vi "fpga.sandbox.test.vi"() -> ()   [LabVIEW 2020]
uses:
  <vilib>/rvi/LocalResourceManager/LocalResourceManager.xnode
  <vilib>/rvi/eio/common/nirviEmuReportErrorAndStop.vi
  <vilib>/rvi/DataTransferAndStorage/Container/Common/niFpgaContainerGetUniqueNameForEmu.vi
  <vilib>/rvi/DataTransferAndStorage/Container/Common/niFpgaContainerSetEmuInfo.vi
  <vilib>/Platform/TimedLoop/XDataNode/wakeup.ctl
  <vilib>/Platform/TimedLoop/XDataNode/XDNodeRunTimeDep.lvlib
  <vilib>/Platform/TimedLoop/XDataNode/nitl_modes.ctl
  <vilib>/Platform/TimedLoop/XDataNode/timing_clust.ctl
  <vilib>/Platform/TimedLoop/XDataNode/XDataNode.xnode
  axi_2_eth_raw.ctl
  <vilib>/rvi/DataTransferAndStorage/Container/XNode/niFpgaContainer.xnode
  <vilib>/rvi/interface/RandomDataEmulation/nirviRandomDataFpgaMultiElementTemplate.vi
  <vilib>/rvi/Memory/Memory_Emulation/niFpgaMemoryEmulationRefIn.vi
  <vilib>/rvi/FIFO/Fifo_Resource/niFpgaFifoEmulationRefIn.vi
  submodules/Market.Data.Bats.Parser/fpga/poc.ip.axi.write.states.ctl
panel:
  in  "ip.Reset":bool
  in  "Reset":bool
  out "Data":T1
  out "i":u16
  out "Numeric":i32
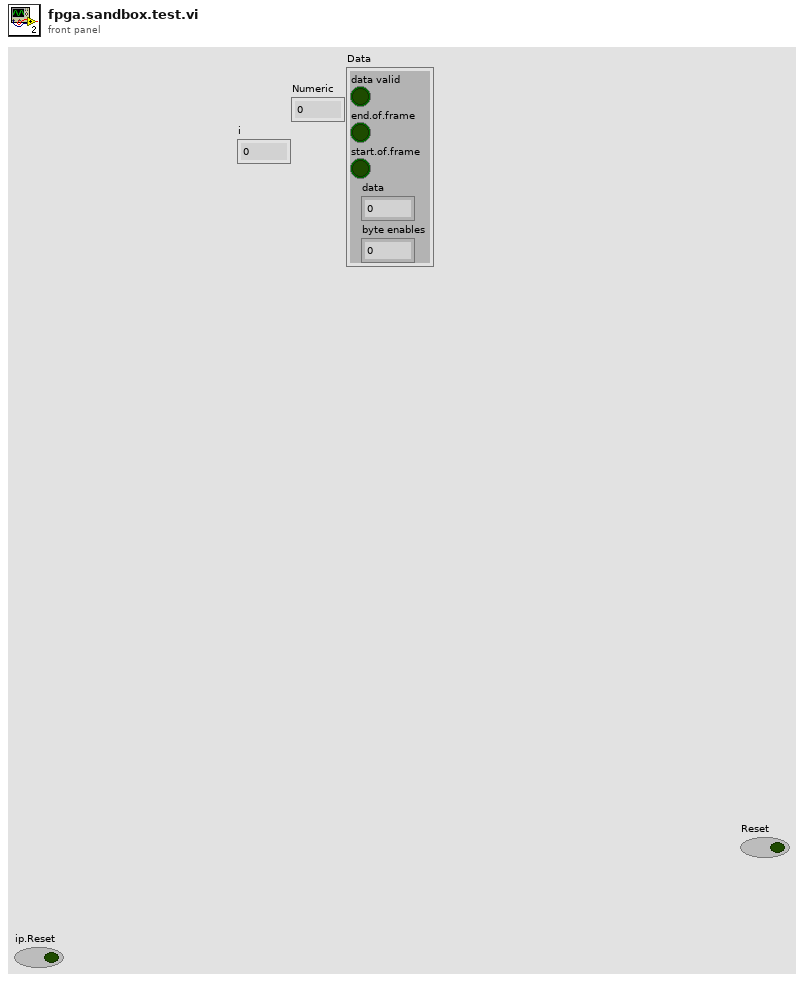
[diagram p1: front panel]
types:
  T1 = cluster{"data valid":bool, "end.of.frame":bool, "start.of.frame":bool, "data":u64, "byte enables":u8}
  T2 = typedef "XDNodeRunTimeDep.lvlib/timing_clust.ctl" = cluster{"Expected End [f-1]":u64, "Actual End [f-1]":u64, "Finished Late? [f-1]":bool, "Expected End [i-1]":u64, "Actual End [i-1]":u64, "Finished Late? [i-1]":bool, "Expected Start [i]":u64, "Actual Start [i]":u64, "Expected Start [f]":u64, "Actual Start [f]":u64, "Source Name":string, "Structure Name":string, "Period":i64, "Deadline":i64, "Offset":i64, "Start":i64, "Priority":i32, "Timeout":i32, "Mode":T3, "Wakeup Reason":T4, "Error":errorcluster, "Source Type":string, "Secondary Source Type":string, "Global End Time":u64, "Global Start Time":u64, "Frame Duration":u64, "Iteration Duration":u64, "Assigned CPU":i32, "I/O Scan Engine Mode":u32}
  T3 = typedef "XDNodeRunTimeDep.lvlib/nitl_modes.ctl" = enum32{"No Change", "Process missed periods, maintain original phase", "Discard missed periods, maintain original phase", "Process missed periods, ignore original phase", "Discard missed periods, ignore original phase"}
  T4 = typedef "XDNodeRunTimeDep.lvlib/wakeup.ctl" = enum32{"Normal", "Aborted", "Asynchronous wakeup", "Timing source error", "Timed loop error", "Timeout"}
  T5 = typedef "axi_2_eth_raw.ctl" = cluster{"data valid":bool, "end.of.frame":bool, "start.of.frame":bool, "data":u64, "byte enables":u8}
  T6 = typedef "poc.ip.axi.write.states.ctl" = enum16{"Wait", "Collect"}
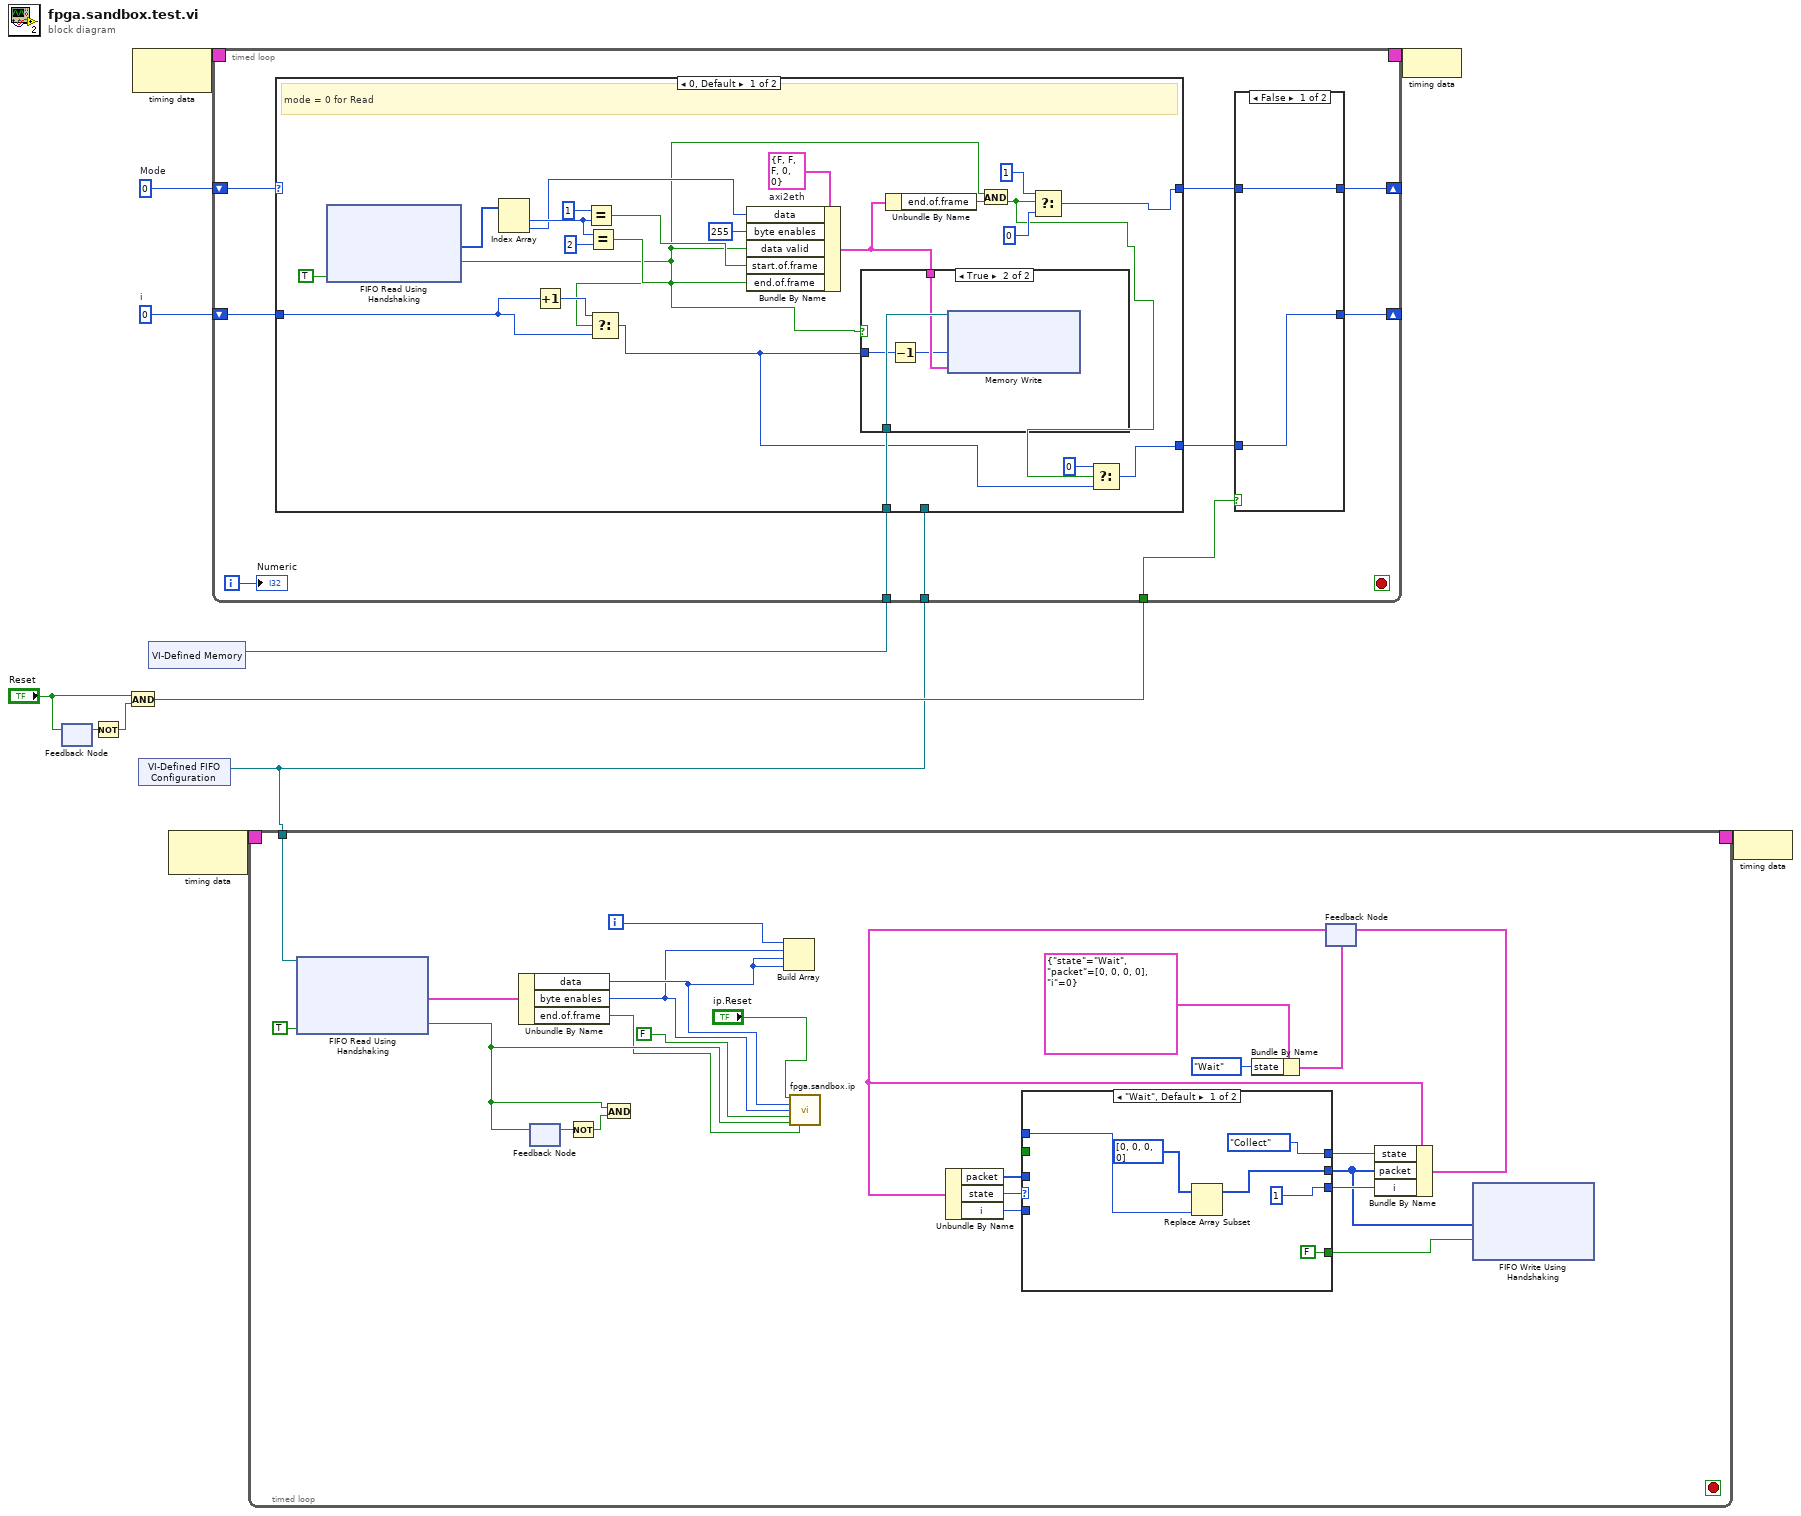
[diagram p0: block diagram]
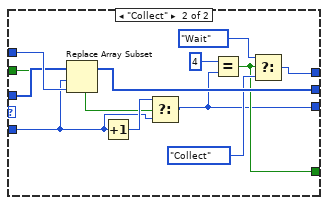
[diagram p2: hidden frame]
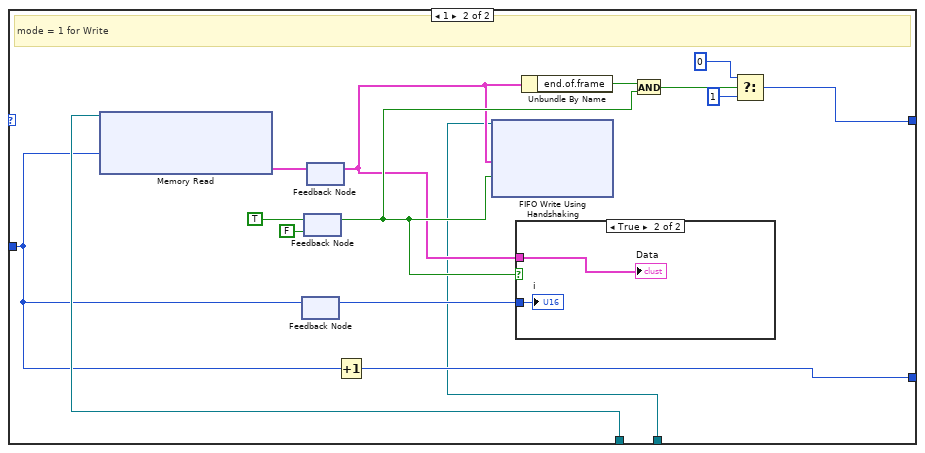
[diagram p4: hidden frame]
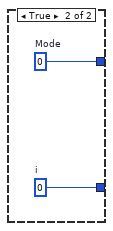
[diagram p6: hidden frame]
diagram:
  w9 = u16 0  # i
  w10 = u8 0  # Mode
  n1 = feedback #1() -> (w8:bool)  [unwired: 1 in]
  n2 = feedback-in #1("Reset") -> ()
  n3 = Not(x=w8) -> (.not. x?=w7:bool)
  n4 = And(x="Reset", y=w7) -> (x .and. y?=w5:bool)
  n5 = node-c288() -> (w12:T2)  [unwired: 1 in]
  n6 = xnode "VI-Defined FIFO Configuration"() -> ("FIFO Out"=w1:refnum<k21>)
  n7 = xnode "VI-Defined Memory"() -> ("Memory Out"=w4:refnum<k21>)
  n8 = node-c288() -> (w3:T2)  [unwired: 1 in]
  n9 = timed-loop {
    timing: w12 -> [_]
    timing-out: [_] -> w11
    tunnel: w1 -> [w15]
    tunnel: w5 -> [w18]
    shift-right: [w22] -> _
    shift-left: w10 -> [w21]
    shift-right: [w20] -> _
    shift-left: w9 -> [w19]
    tunnel: w4 -> [w13]
    i -> [w14]
    stop <- _ stop-if-true
    n10 = case shown="0, Default" w21 {
      tunnel: w19 -> [w34 w52]
      tunnel: w13 -> [w33 w64]
      tunnel: [w26 w58] -> w17
      tunnel: [w28 w61] -> w16
      tunnel: w15 -> [_ w50]
      frame 0, Default {
        w45 = T5 {"data valid"=FALSE, "end.of.frame"=FALSE, "start.of.frame"=FALSE, "data"=0, "byte enables"=0}  # axi2eth
        # "mode = 0 for Read"
        n11 = xnode "FIFO Read Using Handshaking"("Ready for Output"=TRUE) -> ("Element"=w44:u64[], "Output Valid"=w27:bool)  [unwired: 1 in, 1 out]
        n12 = Index Array(array=w44) -> (element #1=w43:u64, element #2=w37:u64)  [unwired: 2 in]
        n13 = Increment(x=w34) -> (x+1=w35:u16)
        n14 = Equal?(x=u64 1, y=w43) -> (x = y?=w39:bool)
        n15 = Equal?(x=w43, y=u64 2) -> (x = y?=w40:bool)
        n16 = Select(t=w35, s=w27, f=w34) -> (s? t:f=w25:u16)
        n17 = Bundle By Name(cluster=w45, "data"=w37, "byte enables"=u8 255 ("number"), "data valid"=w27, "start.of.frame"=w39, "end.of.frame"=w40) -> (w32:T5)
        n18 = case shown="True" w27 {
          tunnel: w33 -> [_ w49]
          tunnel: w32 -> [_ w48]
          tunnel: w25 -> [_ w47]
          frame False {
          }
          frame True {
            n19 = Decrement(x=w47) -> (x-1=w46:u16)
            n20 = xnode "Memory Write"("Address"=w46, "Data"=w48, "Memory In"=w49) -> ()  [unwired: 1 out]
          }
        }
        n21 = Unbundle By Name(w32) -> ("end.of.frame"=w31:bool)
        n22 = And(x=w27, y=w31) -> (x .and. y?=w24:bool)
        n23 = Select(t=u8 1, s=w24, f=u8 0 ("t")) -> (s? t:f=w28:u8)
        n24 = Select(t=u16 0, s=w24, f=w25) -> (s? t:f=w26:u16)
      }
      frame 1 {
        # "mode = 1 for Write"
        n25 = xnode "Memory Read"("Address"=w52, "Memory In"=w64) -> ("Data"=w63:T1)  [unwired: 1 out]
        n26 = feedback-in #2(w52) -> ()
        n27 = feedback #2() -> (w51:u16)  [unwired: 1 in]
        n28 = feedback-in #3(TRUE ("Input Valid")) -> ()
        n29 = feedback #3(FALSE ("Input Valid")) -> (w54:bool)
        n30 = feedback-in #4(w63) -> ()
        n31 = feedback #4() -> (w53:T1)  [unwired: 1 in]
        n32 = Increment(x=w52) -> (x+1=w58:u16)
        n33 = xnode "FIFO Write Using Handshaking"("Element"=w53, "Input Valid"=w54, "FIFO In"=w50) -> ()  [unwired: 2 out]
        n34 = case shown="True" w54 {
          tunnel: w53 -> [_ w66]
          tunnel: w51 -> [_ w65]
          frame False {
          }
          frame True {
            "Data" <- w66
            "i" <- w65
          }
        }
        n35 = Unbundle By Name(w53) -> ("end.of.frame"=w62:bool)
        n36 = And(x=w62, y=w54) -> (x .and. y?=w55:bool)
        n37 = Select(t=u8 0 ("f"), s=w55, f=u8 1) -> (s? t:f=w61:u8)
      }
    }
    n38 = case shown="False" w18 {
      tunnel: [w67 w70] -> w22
      tunnel: [w68 w69] -> w20
      tunnel: w17 -> [w68 _]
      tunnel: w16 -> [w67 _]
      frame False {
      }
      frame True {
        w69 = u16 0  # i
        w70 = u8 0  # Mode
      }
    }
    "Numeric" <- w14
  }
  n39 = timed-loop {
    timing: w3 -> [_]
    timing-out: [_] -> w2
    tunnel: w1 -> [w98]
    i -> [w95]
    stop <- _ stop-if-true
    n40 = xnode "FIFO Read Using Handshaking"("Ready for Output"=TRUE, "FIFO In"=w98) -> ("Element"=w96:T1, "Output Valid"=w74:bool)  [unwired: 1 out]
    n41 = Unbundle By Name(w96) -> ("data"=w77:u64, "byte enables"=w76:u8, "end.of.frame"=w73:bool)
    n42 = feedback #5() -> (w94:bool)  [unwired: 1 in]
    n43 = feedback-in #5(w74) -> ()
    n44 = Not(x=w94) -> (.not. x?=w93:bool)
    n45 = And(x=w74, y=w93) -> ()  [unwired: 1 out]
    n46 = Build Array(w95, w76, w77, w77) -> ()  [unwired: 1 out]
    n47 = call "fpga.sandbox.ip.vi"("ip.reset"="ip.Reset", "TDATA"=w77, "TKEEP"=w76, "TUSER"=FALSE, "TVALID"=w74, "TLAST"=w73) -> ()  [unwired: 10 in]
    n48 = Bundle By Name(cluster=cluster{"state":T6, "packet":u64[], "i":u16} {"state"=enum."Wait", "packet"=[0, 0, 0, 0], "i"=0}, "state"=poc.ip.axi.write.states."Wait" ("Enum")) -> (w88:cluster{"state":T6, "packet":u64[], "i":u16})
    n49 = feedback #6(w88) -> (w87:cluster{"state":T6, "packet":u64[], "i":u16})
    n50 = Unbundle By Name(w87) -> ("packet"=w80:u64[], "state"=w91:T6, "i"=w81:u16)
    n51 = case shown="\"Wait\", Default" w91 {
      tunnel: [FALSE w110] -> w90
      tunnel: [poc.ip.axi.write.states."Collect" ("state") w109] -> w85
      tunnel: [_ w106] -> w84
      tunnel: [w100 w116] -> w83
      tunnel: [u16 1 ("i") w105] -> w82
      tunnel: [w99 w114] -> w79
      tunnel: w81 -> [_ w107]
      tunnel: w80 -> [_ w115]
      frame "Wait", Default {
        n52 = Replace Array Subset(array=u64[] [0, 0, 0, 0] ("packet"), new element=w100) -> (w99:u64[])  [unwired: 1 in]
      }
      frame "Collect" {
        n53 = Replace Array Subset(array=w115, new element=w116, index=w107) -> (w114:u64[])
        n54 = Increment(x=w107) -> (x+1=w108:u16)
        n55 = Select(t=w108, s=w106, f=w107) -> (s? t:f=w105:u16)
        n56 = Equal?(x=u16 4, y=w105) -> (x = y?=w110:bool)
        n57 = Select(t=poc.ip.axi.write.states."Wait" ("Enum"), s=w110, f=poc.ip.axi.write.states."Collect" ("Enum")) -> (s? t:f=w109:T6)
      }
    }
    n58 = Bundle By Name(cluster=w87, "state"=w85, "packet"=w79, "i"=w82) -> (w86:cluster{"state":T6, "packet":u64[], "i":u16})
    n59 = feedback-in #6(w86) -> ()
    n60 = xnode "FIFO Write Using Handshaking"("Element"=w79, "Input Valid"=w90) -> ()  [unwired: 1 in, 2 out]
  }
  n61 = node-c288(w11) -> ()
  n62 = node-c288(w2) -> ()
